vi "calcQmat.vi"(7 "Weighting of Field Point":dbl[](array[numeric]), 8 "error in (no error)":errorcluster, 9 "Sen M":dbl[][][](array[numeric]), 10 "CC Matrix":dbl[][](array[numeric]), 11 "OptCtrl in":refnum<class "OptCtrl.lvclass">) -> (0 "error out":errorcluster, 2 "Q Matrix":dbl[][](array[numeric]), 3 "OptCtrl out":refnum<class "OptCtrl.lvclass">)   [LabVIEW 2016, in "OptCtrl.lvclass"]
doc: "Calculate the Q matrix used in the cost function."
uses:
  OptCtrl.lvclass
  <vilib>/Analysis/baseanly.llb/Real A x B.vi
  <vilib>/Analysis/Matrix/Numeric/Conversions/Array To Matrix - RA2.vi
  <vilib>/Analysis/Matrix/Numeric/Multiply/Multiply - R,RM.vi
  <vilib>/Analysis/Matrix/Numeric/Add/Add - RM,RM.vi
  <vilib>/Analysis/Matrix/Numeric/Conversions/Matrix To Array - RM.vi
  <vilib>/Analysis/Matrix/NI_Matrix.lvlib
  <vilib>/Analysis/NI_AALBase.lvlib
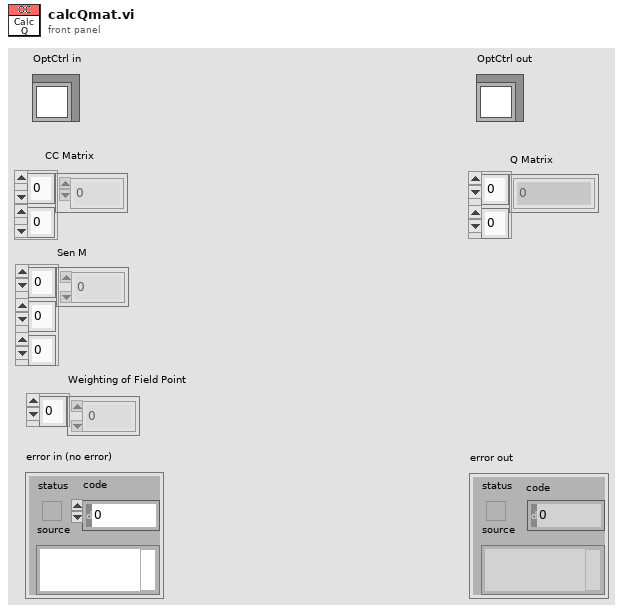
[diagram p1: front panel]
types:
  T1 = typedef "NI_Matrix.lvlib/RealMatrix.ctl" = dbl[][]
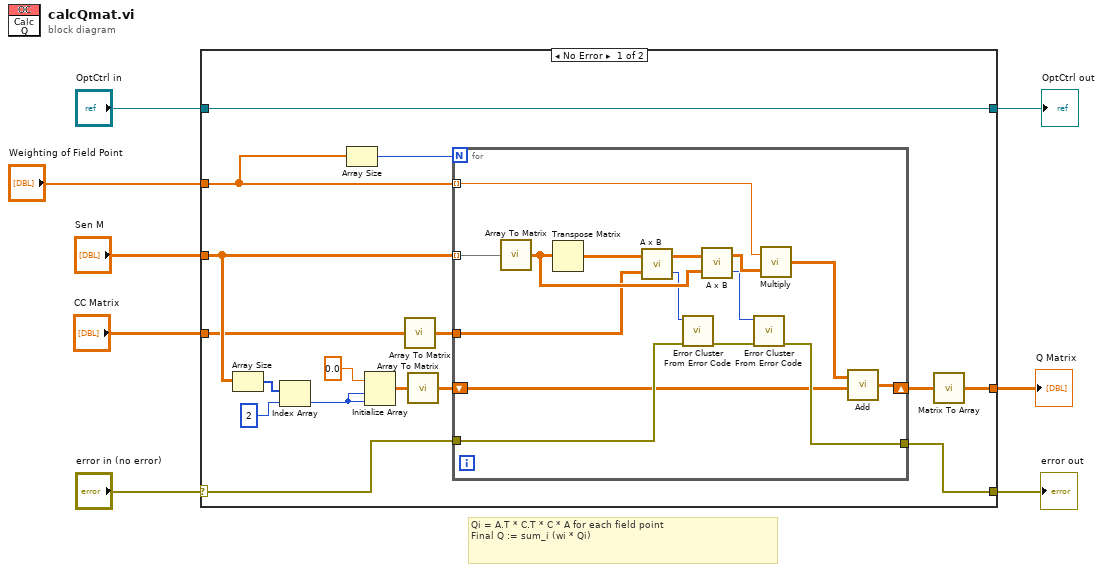
[diagram p0: block diagram]
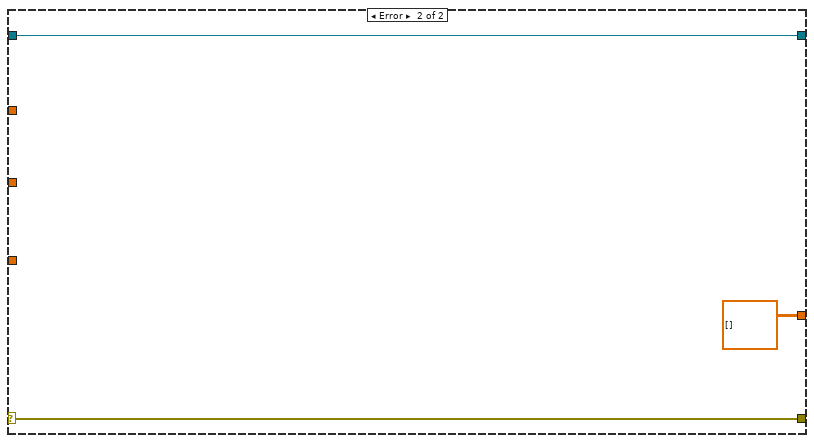
[diagram p2: hidden frame]
diagram:
  # "Qi = A.T * C.T * C * A for each field point\nFinal Q := sum_i (wi * Qi)"
  n1 = case shown="No Error" "error in (no error)" {
    selector: "error in (no error)" -> [w20 w42]
    tunnel: [w19 w42] -> w2
    tunnel: [w24 w41] -> w6
    tunnel: "OptCtrl in" -> [w24 w41]
    tunnel: "Weighting of Field Point" -> [w23 _]
    tunnel: "Sen M" -> [w16 _]
    tunnel: "CC Matrix" -> [w9 _]
    tunnel: [w21 dbl[][] [] ("Real 2D Array")] -> w1
    frame No Error {
      n2 = Array Size(array=w16) -> (size(s)=w15:i32[])
      n3 = Index Array(array=w15, index=2) -> (element=w13:i32)
      n4 = Array Size(array=w23) -> (size(s)=w18:i32)
      n5 = Initialize Array(0.0 ("element"), w13, w13) -> (w11:dbl[][])
      n6 = call-poly <vilib>:"Array To Matrix.vi"("Real 2D Array"=w9) -> ("Real Matrix"=w10:T1)
      n7 = call-poly <vilib>:"Array To Matrix.vi"("Real 2D Array"=w11) -> ("Real Matrix"=w12:T1)
      n8 = for {
        N: w18 -> [_]
        tunnel: w23 -> [w35] mode=indexing
        tunnel: w16 -> [w39] mode=indexing
        shift-right: [w32] -> w22
        shift-left: w12 -> [w26]
        tunnel: w20 -> [w31]
        tunnel: [w27] -> w19
        tunnel: w10 -> [w25]
        n9 = call-poly <vilib>:"Array To Matrix.vi"("Real 2D Array"=w39) -> ("Real Matrix"=w36:T1)
        n10 = Transpose Matrix(1:w36) -> (0:w38:T1)
        n11 = call-poly <vilib>:"A x B.vi"("B"=w25, "A"=w38) -> ("error"=w30:i32, "A x B"=w37:T1)
        n12 = call <vilib>:"Error Cluster From Error Code.vi"("error in (no error)"=w31, "error code (0)"=w30) -> ("error out"=w29:errorcluster)  [unwired: 7 in]
        n13 = call-poly <vilib>:"A x B.vi"("B"=w36, "A"=w37) -> ("error"=w28:i32, "A x B"=w34:T1)
        n14 = call <vilib>:"Error Cluster From Error Code.vi"("error in (no error)"=w29, "error code (0)"=w28) -> ("error out"=w27:errorcluster)  [unwired: 7 in]
        n15 = call-poly <vilib>:"Multiply.vi"("Real Matrix A"=w34, "Real Scalar c"=w35) -> ("c * A"=w33:T1)
        n16 = call-poly <vilib>:"Add.vi"("Real Matrix B"=w26, "Real Matrix A"=w33) -> ("A + B"=w32:T1)
      }
      n17 = call-poly <vilib>:"Matrix To Array.vi"("Real Matrix"=w22) -> ("Real 2D Array"=w21:dbl[][])
    }
    frame Error {
    }
  }
  "error out" <- w2
  "OptCtrl out" <- w6
  "Q Matrix" <- w1
